vi "Create Statement from SQL.vi"(8 "error in (no error)":errorcluster, 9 "Num records":i32, 10 "SQL Dataset":variant[][](array[variant]), 11 "Transaction in":refnum<class "Transaction.lvclass">) -> (0 "error out":errorcluster, 3 "Statement out":refnum<class "Statement.lvclass">)   [LabVIEW 2018, in "Transaction.lvclass"]
uses:
  Transaction.lvclass
  Statement/Statement.lvclass
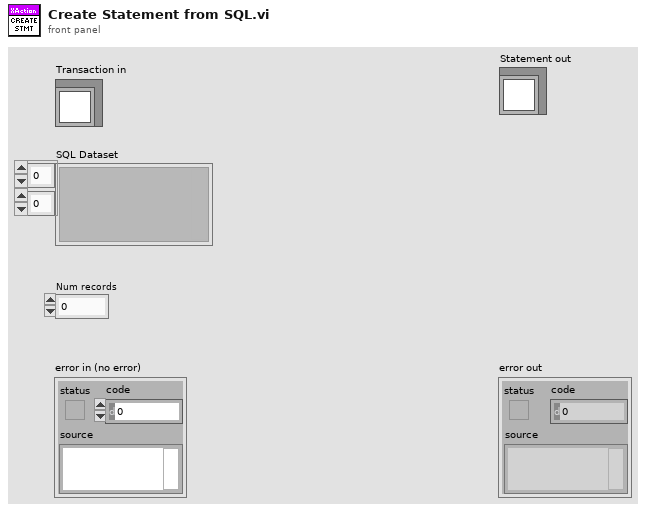
[diagram p1: front panel]
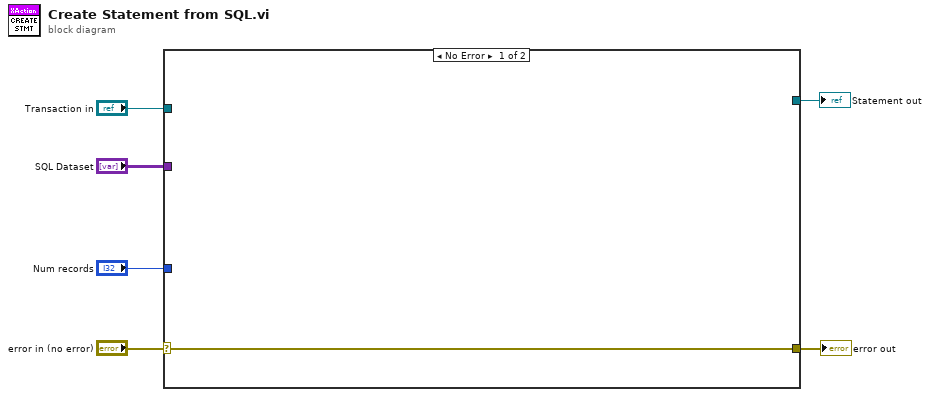
[diagram p0: block diagram]
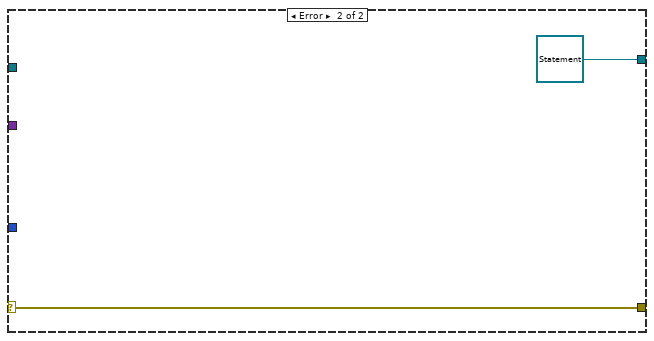
[diagram p2: hidden frame]
diagram:
  n1 = case shown="No Error" "error in (no error)" {
    selector: "error in (no error)" -> [w7 w9]
    tunnel: [w7 w9] -> w5
    tunnel: "Transaction in" -> [_ _]
    tunnel: [_ refnum<class "Statement.lvclass"> refnum ("Statement out")] -> w3
    tunnel: "SQL Dataset" -> [_ _]
    tunnel: "Num records" -> [_ _]
    frame No Error {
    }
    frame Error {
    }
  }
  "error out" <- w5
  "Statement out" <- w3
